vi "escribeListaDePruebas.vi"(8 "error in (no error)":errorcluster, 11 "Dosimetro in":refnum<class "Dosimetro.lvclass">) -> (0 "error out":errorcluster, 3 "Dosimetro out":refnum<class "Dosimetro.lvclass">)   [LabVIEW 2019, in "Dosimetro.lvclass"]
uses:
  Dosimetro.lvclass
  D:/Users/Patricio/Documents/procal-achs/Equipo/Equipo/Equipo.lvclass
  Dosimetro.lvclass/Dosimetro.ctl
  Base de Datos/Base de Datos.lvclass
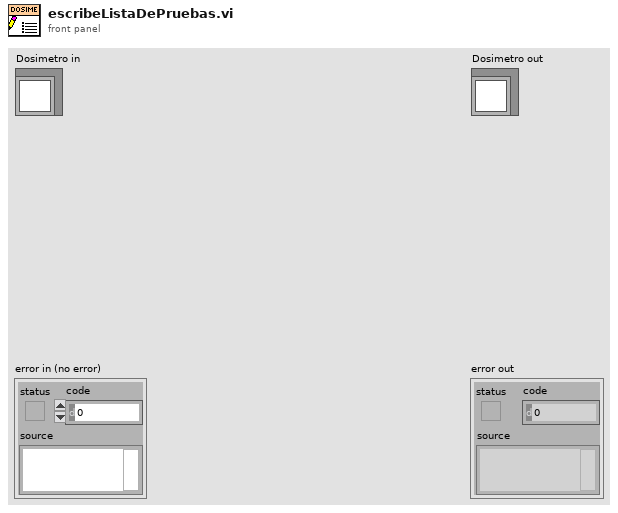
[diagram p1: front panel]
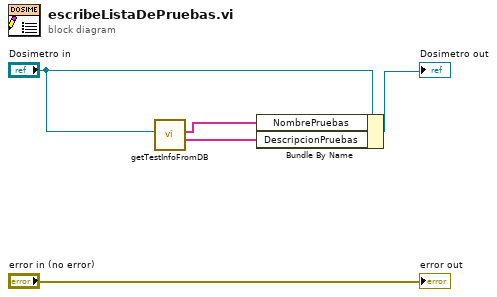
[diagram p0: block diagram]
diagram:
  n1 = call "getTestInfoFromDB.vi"("Equipo.lvclass"="Dosimetro in") -> ("DescripcionPruebas"=w5:string[], "NombrePruebas"=w1:string[])  [unwired: 7 in, 2 out]
  n2 = Bundle By Name(cluster="Dosimetro in", "NombrePruebas"=w1, "DescripcionPruebas"=w5) -> (→"Dosimetro out":refnum<class "Dosimetro.lvclass">)
  "error out" <- "error in (no error)"
